vi "File Flush.vi"(8 "error in":errorcluster, 11 "TDMS in":refnum<class "TDMS.lvclass">) -> (0 "error out":errorcluster, 3 "TDMS out":refnum<class "TDMS.lvclass">)   [LabVIEW 2011, in "TDMS.lvclass"]
uses:
  TDMS.lvclass
  TDMS.lvclass/TDMS.ctl
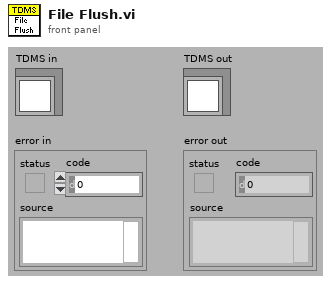
[diagram p1: front panel]
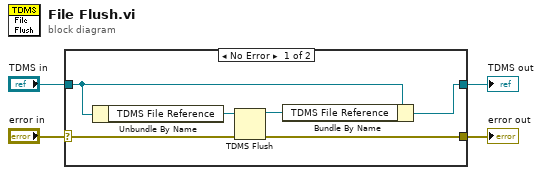
[diagram p0: block diagram]
diagram:
  n1 = case shown="No Error" "error in" {
    selector: "error in" -> [w9 w12]
    tunnel: [w8 w12] -> w3
    tunnel: [w5 w11] -> w1
    tunnel: "TDMS in" -> [w7 w11]
    frame No Error {
      n2 = Unbundle By Name(w7) -> ("TDMS File Reference"=w10:refnum<k34>)
      n3 = TDMS Flush(4:w9, 7:w10) -> (0:w8:errorcluster, 3:w6:refnum<k34>)
      n4 = Bundle By Name(cluster=w7, "TDMS File Reference"=w6) -> (w5:refnum<class "TDMS.lvclass">)
    }
    frame Error {
    }
  }
  "error out" <- w3
  "TDMS out" <- w1
